vi "Stop Data Grid.vi"(8 "error in (no error)":errorcluster, 10 "Delte Datagridview":bool=TRUE, 11 "DataGridView in":refnum<class "DataGridView.lvclass">) -> (0 "error out":errorcluster, 3 "DataGridView out":refnum<class "DataGridView.lvclass">)   [LabVIEW 2013, in "DataGrid.lvlib" / "DataGridView.lvclass"]
doc: "This VI must be called to properly stop the grid, as it unregisters the .net callback events, that otherwise, stay running and lock the classes."
uses:
  DataGridView.lvclass
  DataGridView.lvclass/DataGridView.ctl
  System.Windows.Forms
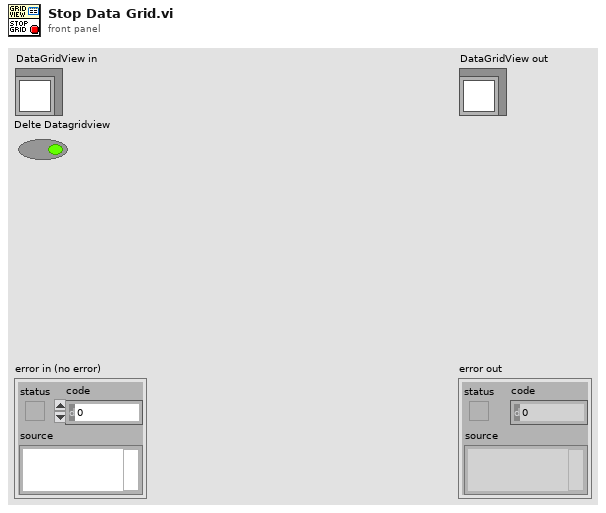
[diagram p1: front panel]
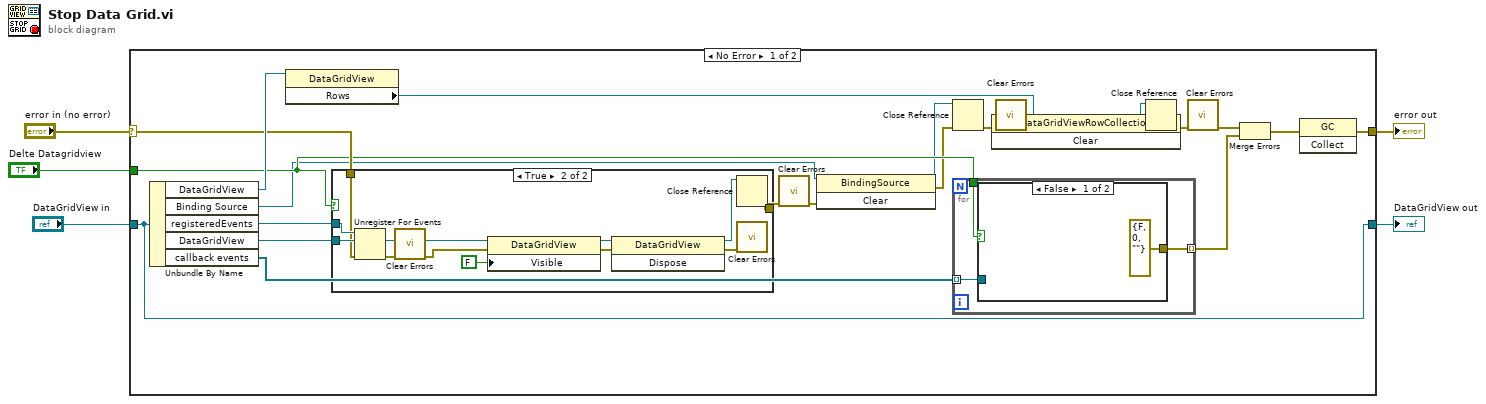
[diagram p0: block diagram]
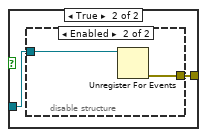
[diagram p3: hidden frame]
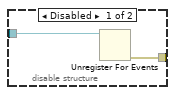
[diagram p4: hidden frame]
diagram:
  n1 = case shown="No Error" "error in (no error)" {
    selector: "error in (no error)" -> [w11 w51]
    tunnel: [w23 w51] -> w4
    tunnel: [w27 w50] -> w2
    tunnel: "DataGridView in" -> [w27 w50]
    tunnel: "Delte Datagridview" -> [w10 _]
    frame No Error {
      n2 = Unbundle By Name(w27) -> ("DataGridView"=w22:refnum<k24>, "Binding Source"=w9:refnum<k24>, "registeredEvents"=w12:refnum<event-registration>, "DataGridView"=w21:refnum<k24>, "callback events"=w26:refnum<k27>[])
      n3 = property class="DataGridView"(reference=w22) -> ("Rows"=w20:refnum<k24>)  [unwired: 1 in, 2 out]
      n4 = case shown="True" w10 {
        tunnel: w21 -> [_ w39]
        tunnel: [w28 w34] -> w17
        tunnel: w12 -> [_ w32]
        tunnel: w11 -> [w28 w29]
        frame False {
        }
        frame True {
          n5 = Unregister For Events(event registration refnum=w32, error in=w29) -> (error out=w31:errorcluster)
          n6 = call <vilib>:"Clear Errors.vi"("error in (no error)"=w31) -> ("error out"=w30:errorcluster)  [unwired: 6 in]
          n7 = property class="DataGridView"(reference=w39, error in=w30, "Visible"=FALSE) -> (reference out=w36:refnum<k24>, error out=w35:errorcluster)
          n8 = invoke class="DataGridView" method="Dispose"(reference=w36, error in=w35) -> (reference out=w38:refnum<k24>, error out=w33:errorcluster)  [unwired: 1 in, 1 out]
          n9 = Close Reference(reference=w38) -> (error out=w34:errorcluster)  [unwired: 1 in]
          n10 = call <vilib>:"Clear Errors.vi"("error in (no error)"=w33) -> ()  [unwired: 6 in, 1 out]
        }
      }
      n11 = call <vilib>:"Clear Errors.vi"("error in (no error)"=w17) -> ("error out"=w19:errorcluster)  [unwired: 6 in]
      n12 = invoke class="BindingSource" method="Clear"(reference=w9, error in=w19) -> (reference out=w8:refnum<k24>, error out=w6:errorcluster)  [unwired: 1 in, 1 out]
      n13 = Close Reference(reference=w8, error in (no error)=w6) -> (error out=w7:errorcluster)
      n14 = for {
        tunnel: w26 -> [w42] mode=indexing
        tunnel: [w41] -> w25 mode=indexing
        tunnel: w10 -> [w40]
        n15 = case shown="False" w40 {
          tunnel: w42 -> [_ w45]
          tunnel: [errorcluster {"status"=FALSE, "code"=0, "source"=""} ("error out") w44] -> w41
          frame False {
          }
          frame True {
            n16 = disable-structure shown="Enabled" {
              disable-tunnel: w45 -> [w47 w49]
              disable-tunnel: [w46 w48] -> w44
              frame Disabled {
                n17 = Unregister For Events(event registration refnum=w47) -> (error out=w46:errorcluster)  [unwired: 1 in]
              }
              frame Enabled {
                n18 = Unregister For Events(event registration refnum=w49) -> (error out=w48:errorcluster)  [unwired: 1 in]
              }
            }
          }
        }
      }
      n19 = call <vilib>:"Clear Errors.vi"("error in (no error)"=w7) -> ("error out"=w18:errorcluster)  [unwired: 6 in]
      n20 = invoke class="DataGridViewRowCollection" method="Clear"(reference=w20, error in=w18) -> (reference out=w14:refnum<k24>, error out=w16:errorcluster)  [unwired: 1 in, 1 out]
      n21 = Close Reference(reference=w14, error in (no error)=w16) -> (error out=w15:errorcluster)
      n22 = call <vilib>:"Clear Errors.vi"("error in (no error)"=w15) -> ("error out"=w13:errorcluster)  [unwired: 6 in]
      n23 = Merge Errors(w13, w25) -> (w24:errorcluster)
      n24 = invoke class="GC" method="Collect"(error in=w24) -> (error out=w23:errorcluster)  [unwired: 2 in, 2 out]
    }
    frame Error {
    }
  }
  "error out" <- w4
  "DataGridView out" <- w2
